vi "Load Config.vi"(8 "error in (no error)":errorcluster, 11 "Config-Sqlite in":refnum<class "Config-Sqlite.lvclass">) -> (0 "error out":errorcluster, 2 "Elements":refnum<class "Config Element.lvclass">[](array[class]), 3 "Config-Sqlite out":refnum<class "Config-Sqlite.lvclass">)   [LabVIEW 2020, in "CDM-Config.lvlib" / "Config-Sqlite.lvclass"]
uses:
  Config-Sqlite.lvclass
  Meta Data.ctl
  Config Element/Config Element.lvclass
  CDM-Config.lvlib
panel:
  out "Array":T2(array[cluster])
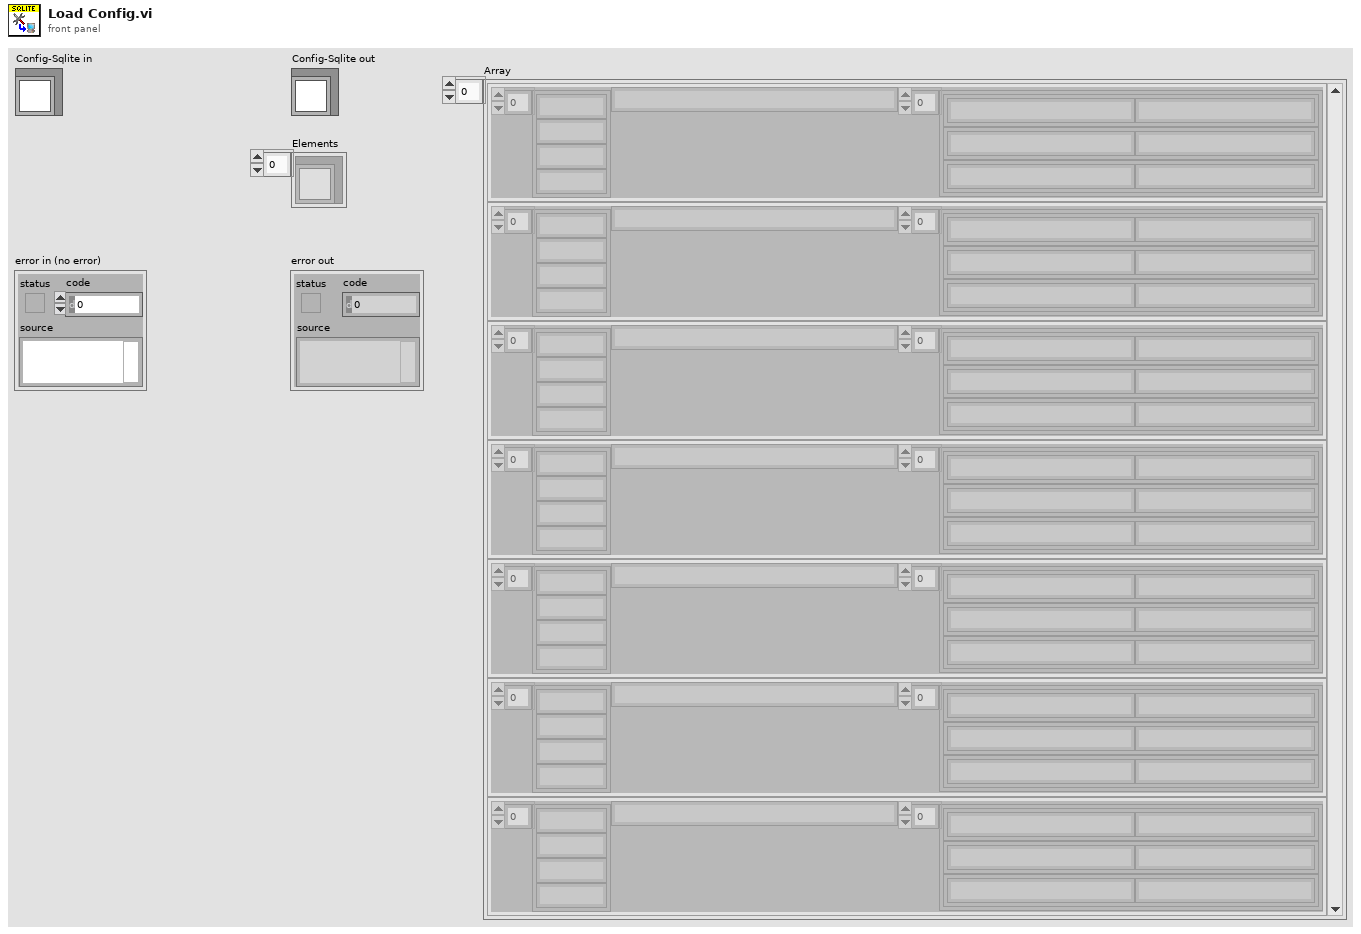
[diagram p1: front panel]
types:
  T1 = typedef "CDM-Config.lvlib/Meta Data.ctl" = cluster{"Name":string, "Value":string}
  T2 = cluster{"Hierarchy":string[], "String Value":string, "Meta Data":T1[]}[]
  T3 = typedef "CDM-Config.lvlib/Config-Sqlite.lvclass/Config.ctl" = cluster{"Row":i32, "Name":string, "Value":string, "Parent":i32, "Meta":T1[]}
  T4 = cluster{"Hierarchy":string[], "String Value":string, "Meta Data":T1[]}
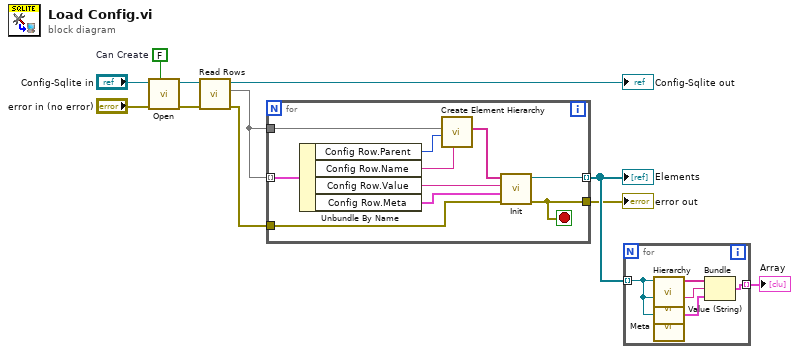
[diagram p0: block diagram]
diagram:
  w5 = FALSE  # Can Create
  n1 = call "Open.vi"("Can Create"=w5, "error in (no error)"="error in (no error)", "Config-Sqlite in"="Config-Sqlite in") -> ("error out"=w8:errorcluster, "Config-Sqlite out"=w10:refnum<class "Config-Sqlite.lvclass">)  [unwired: 7 in]
  n2 = call "Read Rows.vi"("error in (no error)"=w8, "Config-Sqlite in"=w10) -> ("error out"=w7:errorcluster, "Configs"=w6:map{i32, T3}, "Config-Sqlite out"=→"Config-Sqlite out":refnum<class "Config-Sqlite.lvclass">)  [unwired: 7 in]
  n3 = for {
    tunnel: w6 -> [w21] mode=indexing
    tunnel: w7 -> [w18]
    tunnel: w6 -> [w17]
    tunnel: [w13] -> w1
    tunnel: [w12] -> w3 mode=indexing
    stop <- w13 stop-if-true
    n4 = Unbundle By Name(w21) -> ("Config Row.Parent"=w16:i32, "Config Row.Name"=w15:string, "Config Row.Value"=w20:string, "Config Row.Meta"=w19:T1[])
    n5 = call "Create Element Hierarchy.vi"("Name"=w15, "Parent"=w16, "Configs"=w17) -> ("Hierarchy"=w14:string[])  [unwired: 7 in, 1 out]
    n6 = call "Init.vi"("error in (no error)"=w18, "Meta Data"=w19, "Value"=w20, "Hierarchy"=w14) -> ("error out"=w13:errorcluster, "Config Element out"=w12:refnum<class "Config Element.lvclass">)  [unwired: 6 in]
  }
  "error out" <- w1
  "Elements" <- w3
  n7 = for {
    tunnel: w3 -> [w23] mode=indexing
    tunnel: [w24] -> w4 mode=indexing
    n8 = call "Hierarchy.vi"("Config Element in"=w23) -> ("Hierarchy"=w26:string[])  [unwired: 9 in, 1 out]
    n9 = call "Value (String).vi"("Config Element in"=w23) -> ("String Value"=w25:string)  [unwired: 9 in, 1 out]
    n10 = call "Meta.vi"("Config Element in"=w23) -> ("Meta Data"=w22:T1[])  [unwired: 9 in, 1 out]
    n11 = Bundle("Hierarchy"=w26, "String Value"=w25, "Meta Data"=w22) -> (w24:T4)  [unwired: 1 in]
  }
  "Array" <- w4
